vi "Sequence Editor.vi"() -> ()   [LabVIEW 2015, in "Simple Sequence Tools - Editor.lvlib"]
uses:
  Simple Sequence Tools - Editor.lvlib
  Types/UI.PropertiesTypes.ctl
  Types/Main.StateVariables.ctl
  Shared/Types/Channel.Properties.ctl
  Shared/Types/INI.Settings
  Shared/Simple Sequence Tools - Shared.lvlib
panel:
  in  "Sequence":i32[](listbox)
  in  "NIVS.Workspace Event":refnum<event-registration>
  in  "NIVS.Project File Path":path
  in  "Duration Channel":string(combo)
  in  "Skip Channel":string(combo)
  in  "Iteration Information Channel":string(combo)
  in  "Iterations":u32=1 min=1
  in  "Abort Channel":string(combo)
  in  "Step Information Channel":string(combo)
  in  "View":T1=enum."Sequence Properties"
  out "Graph":waveform(dbl)[](graph)
  out "Path":path
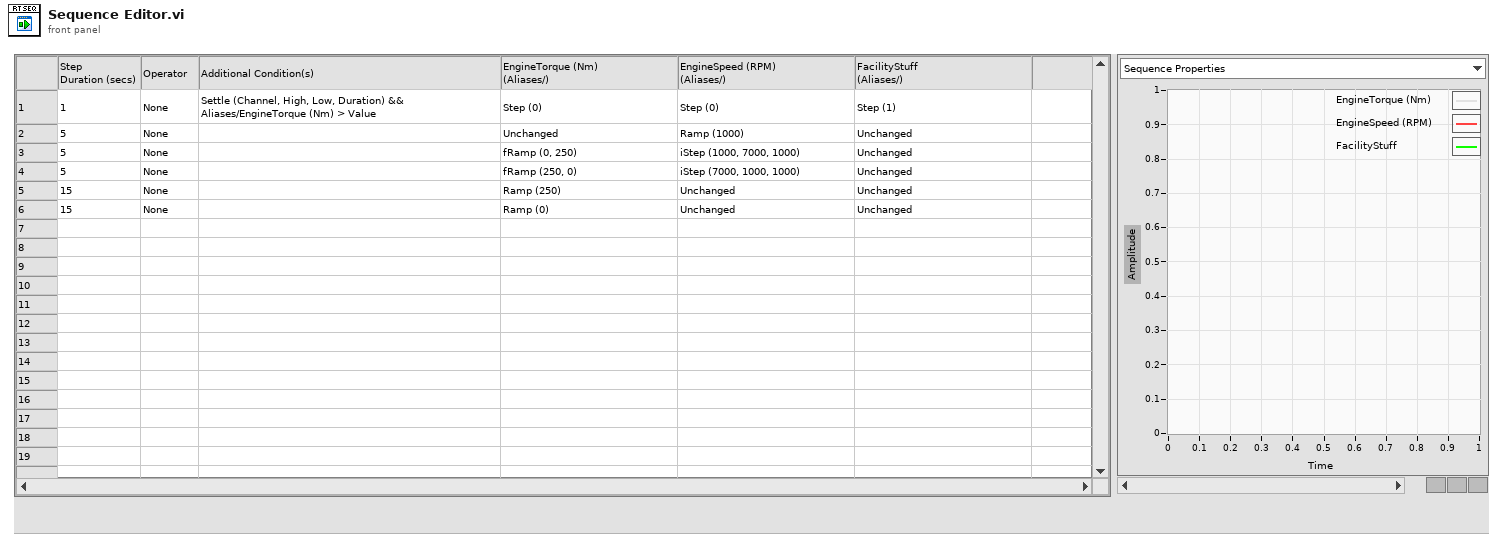
[diagram p1: front panel]
types:
  T1 = typedef "Simple Sequence Tools - Editor.lvlib/UI.PropertiesTypes.ctl" = enum8{"Step Properties", "Sequence Properties"}
  T2 = typedef "Simple Sequence Tools - Editor.lvlib/Main.StateVariables.ctl" = cluster{"Aliases.All":T3[], "Aliases.Outputs":T3[], "UI.Sequence#ofColumns":i32, "SysDef.Path":path, "UI.SequenceRef":refnum<vi>, "UI.StepInformationRef":refnum<vi>, "UI.AbortRef":refnum<vi>, "UI.GraphRef":refnum<vi>, "UI.ViewRef":refnum<vi>, "UI.IterationsRef":refnum<vi>, "UI.IterationInformationRef":refnum<vi>, "INI.Settings":T4, "NIVS.Workspace Event":refnum<event-registration>, "UI.SkipChannel":refnum<vi>, "NIVS.Launched?":bool, "UI.DurationChannel":refnum<vi>}
  T3 = typedef "Simple Sequence Tools - Shared.lvlib/Channel.Properties.ctl" = cluster{"Name":string, "NodePath":string, "ScaleUnits":string}
  T4 = typedef "Simple Sequence Tools - Shared.lvlib/INI.Settings" = cluster{"Build Location":path, "LoggingLocation":path}
  T5 = typedef "LVPoint32TypeDef.ctl" = cluster{"Horizontal":i32, "Vertical":i32}
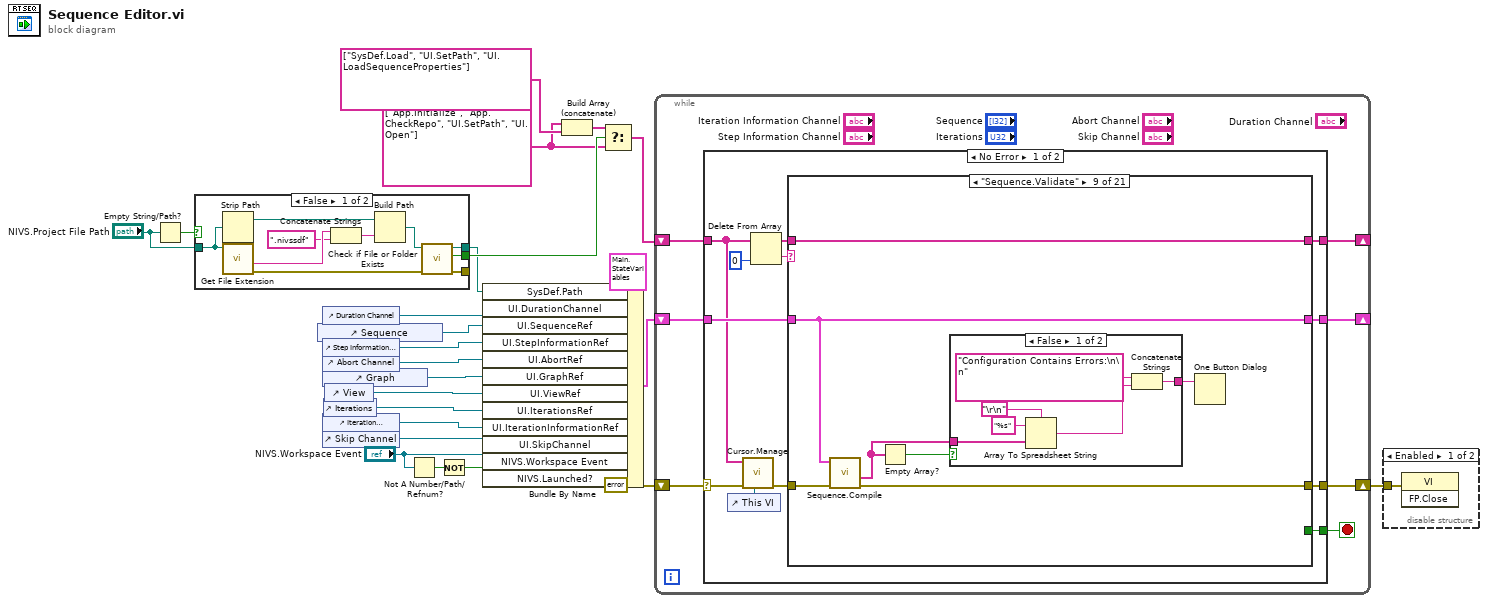
[diagram p0: block diagram]
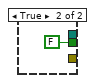
[diagram p2: hidden frame]
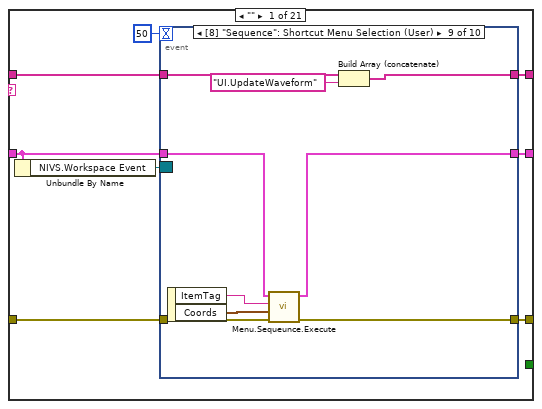
[diagram p4: hidden frame]
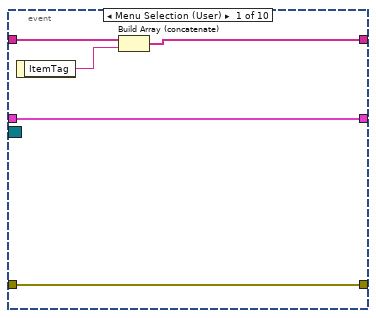
[diagram p5: hidden frame]
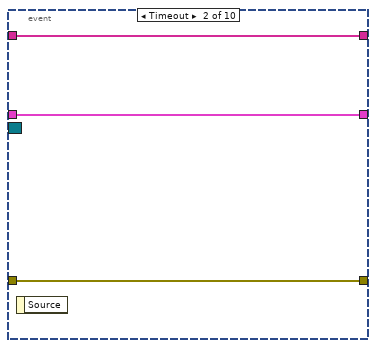
[diagram p6: hidden frame]
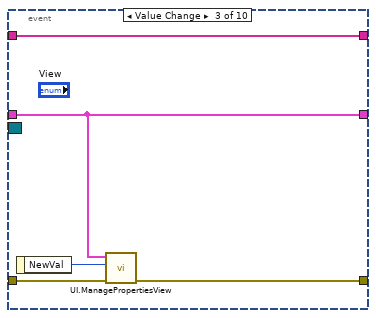
[diagram p7: hidden frame]
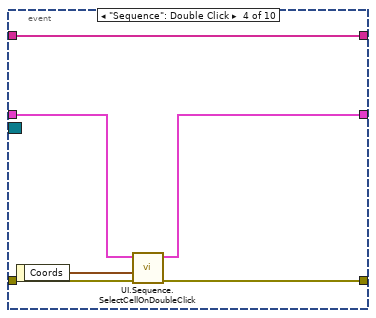
[diagram p8: hidden frame]
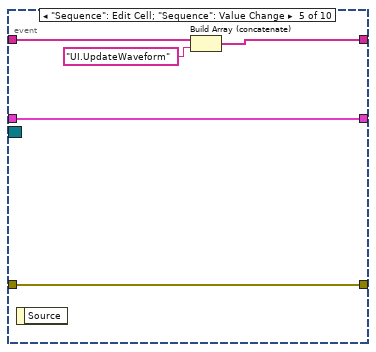
[diagram p9: hidden frame]
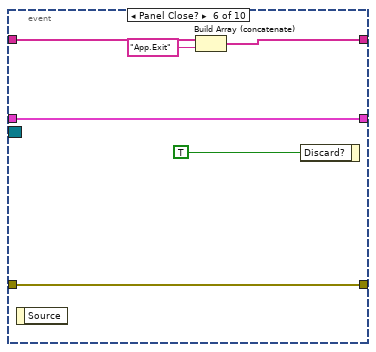
[diagram p10: hidden frame]
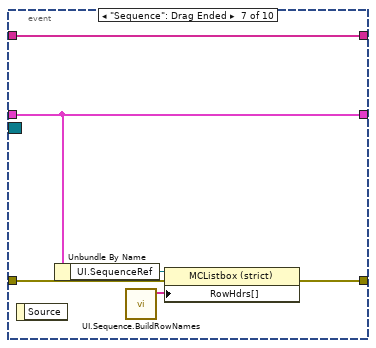
[diagram p11: hidden frame]
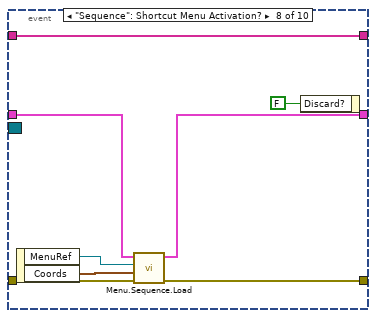
[diagram p12: hidden frame]
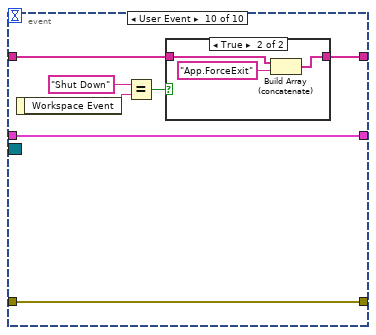
[diagram p13: hidden frame]
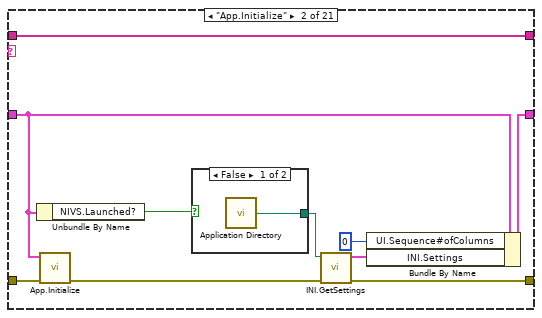
[diagram p15: hidden frame]
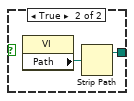
[diagram p16: hidden frame]
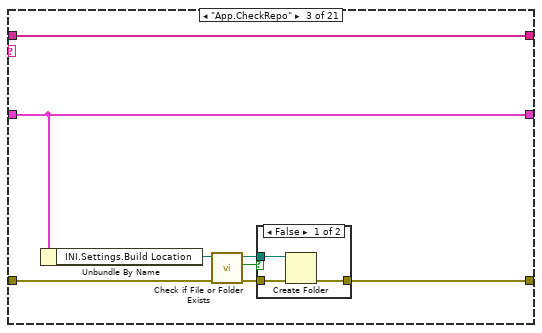
[diagram p17: hidden frame]
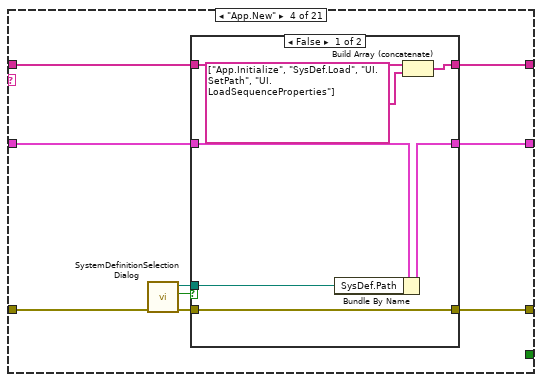
[diagram p19: hidden frame]
diagram:
  w7 = string[] ["App.Initialize", "App.CheckRepo", "UI.SetPath", "UI.Open"]
  n1 = Empty String/Path?(string/path="NIVS.Project File Path") -> (empty?=w11:bool)
  n2 = case shown="False" w11 {
    tunnel: "NIVS.Project File Path" -> [w34 _]
    tunnel: [w27 FALSE ("file or folder exists?")] -> w9
    tunnel: [w26 _] -> _
    tunnel: [w25 _] -> w6
    frame False {
      n3 = Strip Path(path=w34) -> (stripped path=w33:path)  [unwired: 1 out]
      n4 = call <vilib>:"Get File Extension.vi"("file"=w34) -> ("error out"=w28:errorcluster, "filename without extension"=w32:string)  [unwired: 6 in, 3 out]
      n5 = Concatenate Strings(w32, ".nivssdf" ("string")) -> (w30:string)
      n6 = Build Path(base path=w33, name or relative path=w30) -> (appended path=w29:path)
      n7 = call <vilib>:"Check if File or Folder Exists.vi"("error in (no error)"=w28, "path"=w29) -> ("error out"=w26:errorcluster, "file or folder exists?"=w27:bool, "dup path"=w25:path)  [unwired: 7 in]
    }
    frame True {
    }
  }
  n8 = control-ref of="Sequence"() -> (w22:refnum<vi>)
  n9 = control-ref of="Duration Channel"() -> (w1:refnum<vi>)
  n10 = control-ref of="Step Information Channel"() -> (w21:refnum<vi>)
  n11 = control-ref of="Abort Channel"() -> (w20:refnum<vi>)
  n12 = control-ref of="Graph"() -> (w19:refnum<vi>)
  n13 = control-ref of="Iteration Information Channel"() -> (w16:refnum<vi>)
  n14 = control-ref of="Skip Channel"() -> (w14:refnum<vi>)
  n15 = control-ref of="Iterations"() -> (w17:refnum<vi>)
  n16 = control-ref of="View"() -> (w18:refnum<vi>)
  n17 = Not A Number/Path/Refnum?(number/path/refnum="NIVS.Workspace Event") -> (NaN/Path/Refnum?=w4:bool)
  n18 = Not(x=w4) -> (.not. x?=w3:bool)
  n19 = Bundle By Name(cluster=T2 {"Aliases.All"=[], "Aliases.Outputs"=[], "UI.Sequence#ofColumns"=0, "SysDef.Path"=path "", "UI.SequenceRef"=refnum, "UI.StepInformationRef"=refnum, "UI.AbortRef"=refnum, "UI.GraphRef"=refnum, "UI.ViewRef"=refnum, "UI.IterationsRef"=refnum, "UI.IterationInformationRef"=refnum, "INI.Settings"={"Build Location"=path "", "LoggingLocation"=path ""}, "NIVS.Workspace Event"=refnum, "UI.SkipChannel"=refnum, "NIVS.Launched?"=FALSE, "UI.DurationChannel"=refnum}, "SysDef.Path"=w6, "UI.DurationChannel"=w1, "UI.SequenceRef"=w22, "UI.StepInformationRef"=w21, "UI.AbortRef"=w20, "UI.GraphRef"=w19, "UI.ViewRef"=w18, "UI.IterationsRef"=w17, "UI.IterationInformationRef"=w16, "UI.SkipChannel"=w14, "NIVS.Workspace Event"="NIVS.Workspace Event", "NIVS.Launched?"=w3) -> (w2:T2)
  n20 = Build Array (concatenate)(w7, string[] ["SysDef.Load", "UI.SetPath", "UI.LoadSequenceProperties"]) -> (w8:string[])
  n21 = Select(t=w8, s=w9, f=w7) -> (s? t:f=w12:string[])
  n22 = while {
    shift-right: [w41] -> _
    shift-left: w12 -> [w42]
    shift-right: [w39] -> _
    shift-left: w2 -> [w40]
    shift-right: [w37] -> w15
    shift-left: errorcluster {"status"=FALSE, "code"=0, "source"=""} ("error constant") -> [w38]
    stop <- w36 stop-if-true
    n23 = case shown="No Error" w38 {
      selector: w38 -> [w46 w280]
      tunnel: w42 -> [w47 w283]
      tunnel: [w53 w283] -> w41
      tunnel: w40 -> [w51 w282]
      tunnel: [w50 w282] -> w39
      tunnel: [w49 w279] -> w37
      tunnel: [w48 _] -> w36
      frame No Error {
        n24 = control-ref of="This VI"() -> (w43:refnum<vi>)
        n25 = call "Cursor.Manage.vi"("VI reference (current VI)"=w43, "error in (no error)"=w46, "Cmd list"=w47) -> ("error out"=w45:errorcluster)  [unwired: 8 in]
        n26 = Delete From Array(array=w47, index=0) -> (deleted portion=w54:string, array with subset deleted=w52:string[])  [unwired: 1 in]
        n27 = case shown="\"Sequence.Validate\"" w54 {
          tunnel: [w60 w136 w147 w156 w175 w179 w186 w190 w197 w208 w212 w213 w239 w243 w247 w250 w262 w268 w272 w275 w278] -> w53
          tunnel: w52 -> [w59 w136 w147 w157 w175 w179 w186 w190 w197 w208 w212 w214 w239 w243 w248 w249 w262 w268 w272 w275 w278]
          tunnel: w51 -> [w56 w128 w146 w155 w172 w177 w185 w189 w194 w207 w209 w217 w236 w242 w244 w252 w260 w263 w271 w274 w277]
          tunnel: [w62 w131 w146 w158 w171 w177 w185 w189 w194 w207 w209 w215 w235 w242 w244 w252 w260 w265 w271 w274 w277] -> w50
          tunnel: [w57 w133 w141 w159 w173 w178 w184 w188 w195 w205 w211 w218 w237 w240 w245 w253 w261 w266 w269 w273 w276] -> w49
          tunnel: w45 -> [w58 w135 w144 w160 w174 w176 w184 w188 w196 w206 w210 w220 w232 w241 w245 w254 w261 w264 w270 w273 w276]
          tunnel: [_ _ _ _ _ _ w180 TRUE ("T button?") _ _ _ _ _ _ _ _ _ _ _ _ _] -> w48
          frame "" {
            n28 = Unbundle By Name(w56) -> ("NIVS.Workspace Event"=w55:refnum<event-registration>)
            n29 = event shown="[8] \"Sequence\": Shortcut Menu Selection (User)" {
              selector: w55 -> [_ _ _ _ _ _ _ _ _ _]
              dyn-events: _ -> [_ _ _ _ _ _ _ _ _ _]
              timeout: 50 -> [_ _ _ _ _ _ _ _ _ _]
              tunnel: [w64 w70 w75 w81 w83 w88 w98 w106 w108 w116] -> w60
              tunnel: w59 -> [w66 w70 w75 w81 w86 w92 w98 w106 w115 w117]
              tunnel: [w67 w69 w74 w76 w85 w91 w94 w102 w109 w122] -> w62
              tunnel: w56 -> [w67 w69 w74 w77 w85 w91 w94 w101 w110 w122]
              tunnel: [w65 w68 w71 w78 w84 w90 w95 w103 w111 w121] -> w57
              tunnel: w58 -> [w65 w68 w73 w79 w84 w90 w96 w104 w112 w121]
              event Menu Selection (User) {
                n30 = event-data() -> ("ItemTag"=w63:string)  [unwired: 1 in]
                n31 = Build Array (concatenate)(w66, w63) -> (w64:string[])
              }
              event Timeout {
                n32 = event-data() -> ()  [unwired: 1 in, 1 out]
              }
              event Value Change {
                n33 = event-data() -> ("NewVal"=w72:T1)  [unwired: 1 in]
                n34 = call "UI.ManagePropertiesView.vi"("error in (no error)"=w73, "NewVal"=w72, "State Variables"=w74) -> ("error out"=w71:errorcluster)  [unwired: 8 in]
              }
              event "Sequence": Double Click {
                n35 = event-data() -> ("Coords"=w80:T5)  [unwired: 1 in]
                n36 = call "UI.Sequence.SelectCellOnDoubleClick.vi"("error in (no error)"=w79, "Coords"=w80, "State Variables"=w77) -> ("error out"=w78:errorcluster, "State Variables out"=w76:T2)  [unwired: 7 in]
              }
              event "Sequence": Edit Cell; "Sequence": Value Change {
                n37 = event-data() -> ()  [unwired: 1 in, 1 out]
                n38 = Build Array (concatenate)(w86, "UI.UpdateWaveform" ("message")) -> (w83:string[])
              }
              event Panel Close? {
                n39 = event-data() -> ()  [unwired: 1 in, 1 out]
                n40 = Build Array (concatenate)(w92, "App.Exit") -> (w88:string[])
                n41 = event-data("Discard?"=TRUE) -> ()  [unwired: 1 in, 1 out]
              }
              event "Sequence": Drag Ended {
                n42 = event-data() -> ()  [unwired: 1 in, 1 out]
                n43 = Unbundle By Name(w94) -> ("UI.SequenceRef"=w93:refnum<vi>)
                n44 = call "UI.Sequence.BuildRowNames.vi"() -> ("Row Headings"=w97:string[])  [unwired: 11 in]
                n45 = property class="MCListbox (strict)"(reference=w93, error in=w96, "RowHdrs[]"=w97) -> (error out=w95:errorcluster)  [unwired: 1 out]
              }
              event "Sequence": Shortcut Menu Activation? {
                n46 = event-data() -> ("MenuRef"=w99:refnum<k9>, "Coords"=w100:T5)  [unwired: 1 in]
                n47 = call "Menu.Sequence.Load.vi"("error in (no error)"=w104, "Coords"=w100, "MenuRef"=w99, "State Variables"=w101) -> ("error out"=w103:errorcluster, "State Variables out"=w102:T2)  [unwired: 6 in]
                n48 = event-data("Discard?"=FALSE) -> ()  [unwired: 1 in, 1 out]
              }
              event "Sequence": Shortcut Menu Selection (User) {
                n49 = event-data() -> ("ItemTag"=w114:string, "Coords"=w113:T5)  [unwired: 1 in]
                n50 = call "Menu.Sequeunce.Execute.vi"("error in (no error)"=w112, "Coords"=w113, "ItemPath"=w114, "State Variables"=w110) -> ("error out"=w111:errorcluster, "State Variables out"=w109:T2)  [unwired: 6 in]
                n51 = Build Array (concatenate)(w115, "UI.UpdateWaveform" ("message")) -> (w108:string[])
              }
              event User Event {
                n52 = event-data() -> ("Workspace Event"=w119:string)  [unwired: 1 in]
                n53 = Equal?(x="Shut Down" ("y"), y=w119) -> (x = y?=w118:bool)
                n54 = case shown="True" w118 {
                  tunnel: w117 -> [w123 w125]
                  tunnel: [w123 w124] -> w116
                  frame False {
                  }
                  frame True {
                    n55 = Build Array (concatenate)(w125, "App.ForceExit") -> (w124:string[])
                  }
                }
              }
            }
          }
          frame "App.Initialize" {
            n56 = Unbundle By Name(w128) -> ("NIVS.Launched?"=w127:bool)
            n57 = call "App.Initialize.vi"("error in (no error)"=w135, "Start Variables"=w128) -> ("error out"=w134:errorcluster)  [unwired: 9 in]
            n58 = case shown="False" w127 {
              tunnel: [w137 w138] -> w130
              frame False {
                n59 = call <vilib>:"Application Directory.vi"() -> ("Application Directory"=w137:path)
              }
              frame True {
                n60 = property class="VI"() -> ("Path"=w139:path)  [unwired: 2 in, 2 out]
                n61 = Strip Path(path=w139) -> (stripped path=w138:path)  [unwired: 1 out]
              }
            }
            n62 = call "INI.GetSettings.vi"("error in (no error)"=w134, "INI Folder Location"=w130) -> ("error out"=w133:errorcluster, "INI.Settings"=w132:T4)  [unwired: 8 in]
            n63 = Bundle By Name(cluster=w128, "UI.Sequence#ofColumns"=0, "INI.Settings"=w132) -> (w131:T2)
          }
          frame "App.CheckRepo" {
            n64 = Unbundle By Name(w146) -> ("INI.Settings.Build Location"=w145:path)
            n65 = call <vilib>:"Check if File or Folder Exists.vi"("error in (no error)"=w144, "path"=w145) -> ("error out"=w142:errorcluster, "file or folder exists?"=w140:bool, "dup path"=w143:path)  [unwired: 7 in]
            n66 = case shown="False" w140 {
              tunnel: w143 -> [w150 _]
              tunnel: w142 -> [w149 w151]
              tunnel: [w148 w151] -> w141
              frame False {
                n67 = Create Folder(path (use dialog)=w150, error in=w149) -> (error out=w148:errorcluster)  [unwired: 1 in, 2 out]
              }
              frame True {
              }
            }
          }
          frame "App.New" {
            n68 = call "SystemDefinitionSelectionDialog.vi"("error in (no error)"=w160) -> ("error out"=w154:errorcluster, "cancelled"=w153:bool, "selected path"=w152:path)  [unwired: 8 in]
            n69 = case shown="False" w153 {
              tunnel: w154 -> [w167 w169]
              tunnel: [w167 w169] -> w159
              tunnel: w155 -> [w161 w170]
              tunnel: [w166 w170] -> w158
              tunnel: w152 -> [w165 _]
              tunnel: [w164 w168] -> w156
              tunnel: w157 -> [w162 w168]
              frame False {
                n70 = Bundle By Name(cluster=w161, "SysDef.Path"=w165) -> (w166:T2)
                n71 = Build Array (concatenate)(w162, string[] ["App.Initialize", "SysDef.Load", "UI.SetPath", "UI.LoadSequenceProperties"]) -> (w164:string[])
              }
              frame True {
              }
            }
          }
          frame "App.Open" {
            n72 = call "App.Open.vi"("error in (no error)"=w174, "State Variables"=w172) -> ("error out"=w173:errorcluster, "State Variables out"=w171:T2)  [unwired: 8 in]
          }
          frame "App.Save" {
            n73 = call "App.Save.vi"("error in (no error)"=w176, "State Variables"=w177) -> ("error out"=w178:errorcluster)  [unwired: 9 in]
          }
          frame "App.Exit" {
            n74 = Two Button Dialog(message="Any unsaved and unbuilt changes will be lost.  Are you sure you want to exit?", 1:"No" ("F button name (\"Cancel\")"), 2:"Yes" ("T button name (\"OK\")")) -> (T button?=w180:bool)
          }
          frame "App.ForceExit" {
          }
          frame "Sequence.Validate" {
            n75 = call "Sequence.Compile.vi"("error in (no error)"=w196, "State Variables"=w194) -> ("error out"=w195:errorcluster, "Warnings"=w191:string[])  [unwired: 7 in, 1 out]
            n76 = Empty Array?(array=w191) -> (empty?=w193:bool)
            n77 = case shown="False" w193 {
              tunnel: [w201 "Configuration Valid"] -> w192
              tunnel: w191 -> [w202 _]
              frame False {
                n78 = Array To Spreadsheet String(delimiter (Tab)="\r\n", array=w202, 3:"%s" ("format string")) -> (spreadsheet string=w200:string)
                n79 = Concatenate Strings("Configuration Contains Errors:\n\n", w200) -> (w201:string)
              }
              frame True {
              }
            }
            n80 = One Button Dialog(message=w192) -> ()  [unwired: 1 in, 1 out]
          }
          frame "Sequence.Preview" {
            n81 = call "Sequence.Preview.vi"("error in (no error)"=w206, "State Variables"=w207) -> ("error out"=w205:errorcluster)  [unwired: 9 in]
          }
          frame "Sequence.Build" {
            n82 = call "Sequence.Build.vi"("error in (no error)"=w210, "State Variables"=w209) -> ("error out"=w211:errorcluster)  [unwired: 9 in]
          }
          frame "SysDef.New" {
            n83 = call "SystemDefinitionSelectionDialog.vi"("error in (no error)"=w220) -> ("error out"=w221:errorcluster, "cancelled"=w219:bool, "selected path"=w216:path)  [unwired: 8 in]
            n84 = case shown="False" w219 {
              tunnel: w221 -> [w228 w230]
              tunnel: [w228 w230] -> w218
              tunnel: w217 -> [w227 w231]
              tunnel: [w226 w231] -> w215
              tunnel: w216 -> [w225 _]
              tunnel: [w224 w229] -> w213
              tunnel: w214 -> [w222 w229]
              frame False {
                n85 = Bundle By Name(cluster=w227, "SysDef.Path"=w225) -> (w226:T2)
                n86 = Build Array (concatenate)(w222, string[] ["SysDef.Load", "UI.SetPath", "UI.LoadSequenceProperties"]) -> (w224:string[])
              }
              frame True {
              }
            }
          }
          frame "SysDef.Load" {
            n87 = Unbundle By Name(w236) -> ("SysDef.Path"=w238:path)
            n88 = call "LoadSystemDefinition.vi"("error in (no error)"=w232, "SysDef.Path"=w238) -> ("error out"=w237:errorcluster, "Aliases.Outputs"=w233:T3[], "Aliases.All"=w234:T3[])  [unwired: 7 in]
            n89 = Bundle By Name(cluster=w236, "Aliases.All"=w234, "Aliases.Outputs"=w233) -> (w235:T2)
          }
          frame "SysDef.Edit" {
            n90 = call "SysDef.Edit.vi"("error in (no error)"=w241, "State Variables"=w242) -> ("error out"=w240:errorcluster)  [unwired: 9 in]
          }
          frame "SysDef.Refresh" {
            n91 = Build Array (concatenate)(w248, string[] ["SysDef.Load", "UI.SetPath", "UI.LoadSequenceProperties"]) -> (w247:string[])
          }
          frame "Steps.GenerateMultiple" {
            n92 = call "Dialog.MassStepGeneration.vi"("error in (no error)"=w254, "State Variables"=w252) -> ("error out"=w253:errorcluster, "Canceled"=w251:bool)  [unwired: 8 in]
            n93 = case shown="False" w251 {
              tunnel: [w256 w258] -> w250
              tunnel: w249 -> [w257 w258]
              frame False {
                n94 = Build Array (concatenate)(w257, "UI.UpdateWaveform" ("message")) -> (w256:string[])
              }
              frame True {
              }
            }
          }
          frame "UI.SetPath" {
            n95 = Unbundle By Name(w260) -> ("SysDef.Path"=→"Path":path)
          }
          frame "UI.UpdateWaveform" {
            n96 = call "UI.UpdateWaveform.vi"("error in (no error)"=w264, "State Variables"=w263) -> ("error out"=w266:errorcluster, "Wavefrom"=→"Graph":waveform(dbl)[], "State Variables out"=w265:T2)  [unwired: 7 in]
          }
          frame "UI.LoadSequenceProperties" {
            n97 = call "UI.LoadComboBoxes.vi"("error in (no error)"=w270, "State Variables"=w271) -> ("error out"=w269:errorcluster)  [unwired: 9 in]
          }
          frame "UI.Open" {
            n98 = invoke class="VI" method="FP.Open"() -> ()  [unwired: 5 in, 5 out]
          }
          frame Default {
          }
        }
      }
      frame Error {
        n99 = call <vilib>:"Simple Error Handler.vi"("error in (no error)"=w280) -> ("error out"=w281:errorcluster)  [unwired: 4 in, 4 out]
        n100 = call <vilib>:"Clear Errors.vi"("error in (no error)"=w281) -> ("error out"=w279:errorcluster)  [unwired: 5 in, 1 out]
      }
    }
  }
  n101 = disable-structure shown="Enabled" {
    disable-tunnel: w15 -> [w284 _]
    frame Enabled {
      n102 = invoke class="VI" method="FP.Close"(error in=w284) -> ()  [unwired: 2 in, 3 out]
    }
    frame Disabled {
    }
  }
